vi "Go To RGB Color Now.vi"(7 "I2C Channel (0)":u8, 8 "Error In":errorcluster, 9 "Color":u32(colorbox), 10 "I2C Slave Address (0)":u8, 11 "LINX Resource":T1) -> (0 "Error Out":errorcluster, 3 "LINX Resource":T1)   [LabVIEW 2020, in "LMH-LINX.lvlib" / "BlinkM.lvlib"]
doc: "Set the BlinkM's RGB color immediatly."
uses:
  BlinkM.lvlib
  LMH-LINX.lvlib
  Private/Type Defs/Platform.ctl
  Private/Type Defs/Interface.ctl
  Private/Type Defs/LINX Ref.ctl
  Private/Device/Type Defs/Channels.ctl
  Private/Device/Type Defs/TCP Config.ctl
  Private/Device/Device.lvlib
  Private/Device/Type Defs/LINX Device Config.ctl
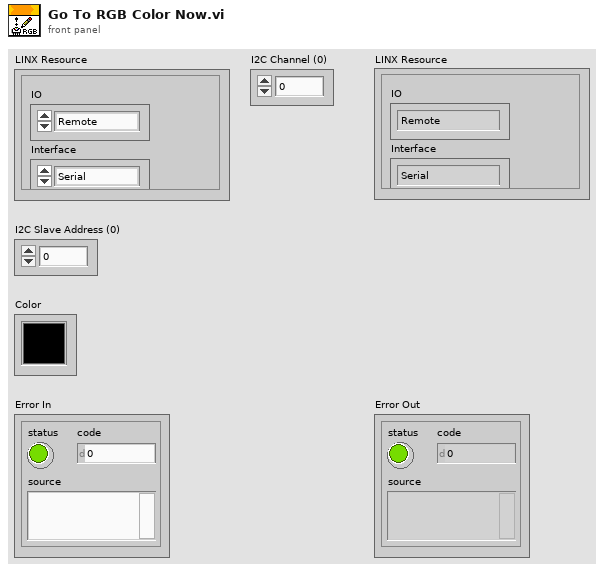
[diagram p1: front panel]
types:
  T1 = typedef "LMH-LINX.lvlib/LINX Ref.ctl" = cluster{"IO":T2, "Interface":T3, "LINX Device Config":T4}
  T2 = typedef "LMH-LINX.lvlib/Platform.ctl" = enum16{"Remote", "Local"}
  T3 = typedef "LMH-LINX.lvlib/Interface.ctl" = enum16{"Serial", "TCP"}
  T4 = typedef "Device.lvlib/LINX Device Config.ctl" = cluster{"Interface":T3, "COM Port":refnum<visa-resource-name>, "TCP Configuration":T5, "Device Family":u8, "Device ID":u8, "Device Name":string, "TCP Ref":refnum<k5>, "Channels":T6}
  T5 = typedef "Device.lvlib/TCP Config.ctl" = cluster{"IP Address":string, "Port":u16}
  T6 = typedef "LMH-LINX.lvlib/Channels.ctl" = cluster{"DI":u8[], "DO":u8[], "AI":u8[], "AO":u8[], "PWM":u8[], "QE":u8[], "UART":u8[], "I2C 2":u8[], "SPI":u8[], "CAN":u8[], "Servo":u8[], "AI Ref (V)":dbl, "AI Resolution (Bits)":u8, "AO Ref (V)":dbl, "AO Resolution (Bits)":u8}
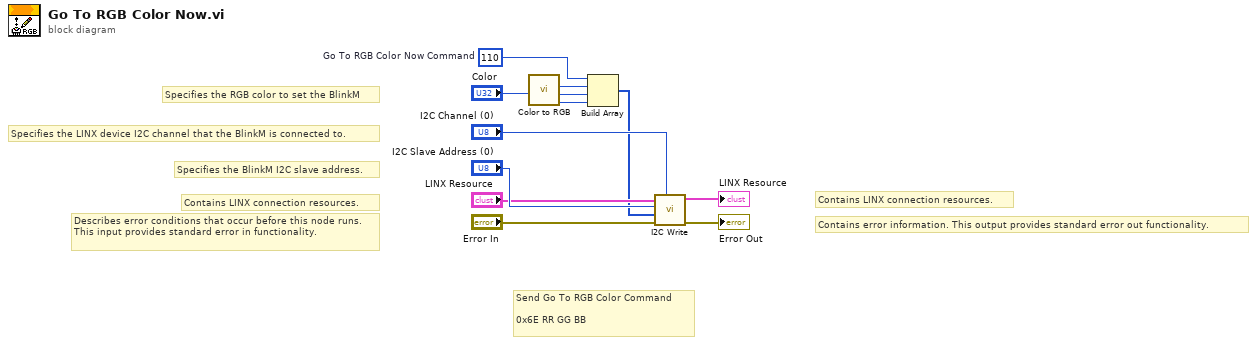
[diagram p0: block diagram]
diagram:
  w5 = u8 110  # Go To RGB Color Now Command
  # "Specifies the RGB color to set the BlinkM"
  # "Specifies the BlinkM I2C slave address."
  # "Specifies the LINX device I2C channel that the BlinkM is connected to."
  # "Contains LINX connection resources."
  # "Contains error information. This output provides standard error out functionality."
  # "Contains LINX connection resources."
  # "Describes error conditions that occur before this node runs. This input provides standard error in functionality."
  # "Send Go To RGB Color Command\n\n0x6E RR GG BB"
  n1 = call <vilib>:"Color to RGB.vi"("Color"="Color") -> ("R"=w4:u8, "G"=w3:u8, "B"=w2:u8)  [unwired: 1 out]
  n2 = Build Array(w5, w4, w3, w2) -> (w1:u8[])
  n3 = call "I2C Write.vi"("I2C Channel"="I2C Channel (0)", "Error In"="Error In", "Data"=w1, "I2C Slave Address (0)"="I2C Slave Address (0)", "LINX Resource"="LINX Resource") -> ("Error Out"=→"Error Out":errorcluster, "LINX Resource"=→"LINX Resource":T1)  [unwired: 5 in]
